vi "Write Logger.vi"(8 "error in (no error)":errorcluster, 10 "Logger":refnum<class "Logger Interface.lvclass">, 11 "Log Producer in":refnum<class "Log Producer.lvclass">) -> (0 "error out":errorcluster, 3 "Log Producer out":refnum<class "Log Producer.lvclass">)   [LabVIEW 2023, in "Ballard MIL-STD-1553 Engine Support.lvlib" / "Implementation.lvlib" / "Word Logging.lvlib" / "Log Producer.lvclass"]
uses:
  Log Producer.lvclass
  Logger Interface/Logger Interface.lvclass
  Log Producer.lvclass/Log Producer.ctl
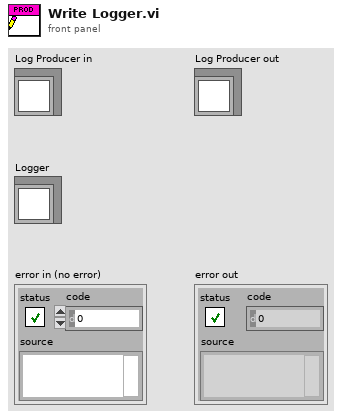
[diagram p1: front panel]
types:
  T1 = typedef "Ballard MIL-STD-1553 Engine Support.lvlib/Implementation.lvlib/Word Logging.lvlib/Logger Data Reference.ctl" = refnum<data-value>
  T2 = cluster{"Logger":refnum<class "Logger Interface.lvclass">}
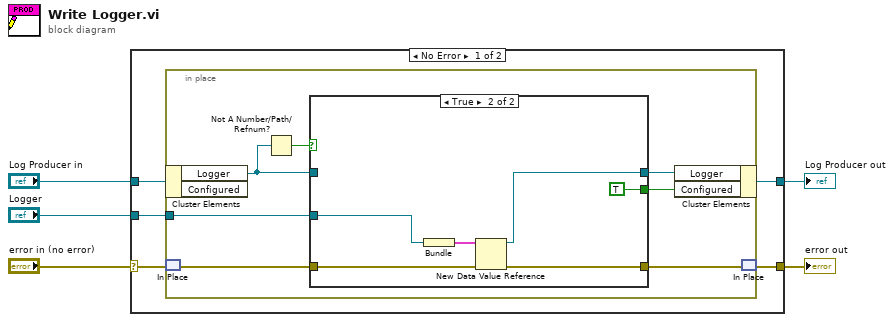
[diagram p0: block diagram]
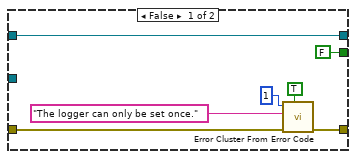
[diagram p2: hidden frame]
diagram:
  n1 = case shown="No Error" "error in (no error)" {
    selector: "error in (no error)" -> [w10 w31]
    tunnel: [w9 w31] -> w4
    tunnel: [w7 w32] -> w2
    tunnel: "Log Producer in" -> [w8 w32]
    tunnel: "Logger" -> [w6 _]
    frame No Error {
      n2 = in-place {
        in-place-border: w6 -> [w16]
        n3 = in-place-cluster #1(w8) -> ("Logger"=w13:T1)  [unwired: 1 out]
        n4 = in-place-match #2(w10) -> (w15:errorcluster)
        n5 = Not A Number/Path/Refnum?(number/path/refnum=w13) -> (NaN/Path/Refnum?=w12:bool)
        n6 = case shown="True" w12 {
          tunnel: [w19 w30] -> w17
          tunnel: w16 -> [_ w27]
          tunnel: w15 -> [w23 w29]
          tunnel: [w24 w28] -> w14
          tunnel: w13 -> [w19 _]
          tunnel: [FALSE TRUE] -> w11
          frame False {
            n7 = call <vilib>:"Error Cluster From Error Code.vi"("show call chain? (False)"=TRUE, "error in (no error)"=w23, "error message (\"\")"="The logger can only be set once." ("error message (\"\")"), "error code (0)"=1) -> ("error out"=w24:errorcluster)  [unwired: 5 in]
          }
          frame True {
            n8 = Bundle("Logger"=w27) -> (w26:T2)  [unwired: 1 in]
            n9 = New Data Value Reference(data value=w26, error in=w29) -> (data value reference=w30:refnum<data-value>, error out=w28:errorcluster)
          }
        }
        n10 = in-place-cluster #1("Logger"=w17, "Configured"=w11) -> (w7:refnum<class "Log Producer.lvclass">)
        n11 = in-place-match #2(w14) -> (w9:errorcluster)
      }
    }
    frame Error {
    }
  }
  "error out" <- w4
  "Log Producer out" <- w2
